vi "CheckWhetherSendMissions.vi"(10 "Mission Notifiers":T1, 11 "NotifierReff":T2) -> (2 "Send obstacles?":bool, 3 "Send missions?":bool)   [LabVIEW 2013]
doc: "This VI checks whether last the mission and obstacle ID held by the OCU matches that of the boat. If not, it signals that the missions need to be sent to the OCU to line the boat and OCU up again.\n\nEric Schneider, August 2014"
uses:
  Data/TypeDefs/Notifiers.ctl
  Data/TypeDefs/UTM Location.ctl
  Data/TypeDefs/Sail Set Suggestions.ctl
  Data/TypeDefs/Rudder Set Suggestions.ctl
  Data/TypeDefs/OverrideInformation.ctl
  Data/TypeDefs/OverrideMode.ctl
  Data/TypeDefs/MotorSetup.ctl
  Data/TypeDefs/DynamixelSetupInfo.ctl
  Data/TypeDefs/AirmarStatus.ctl
  Data/TypeDefs/HardwareOnline.ctl
  Data/TypeDefs/DynamixelCycleTracker.ctl
  Data/TypeDefs/RC Input Values.ctl
  Classes/Waypoint/Waypoint.lvclass
  Data/TypeDefs/MissionNotifiers.ctl
  Classes/Missions/GenericMission/GenericMission.lvclass
  Classes/Obstacle/Obstacle.lvclass
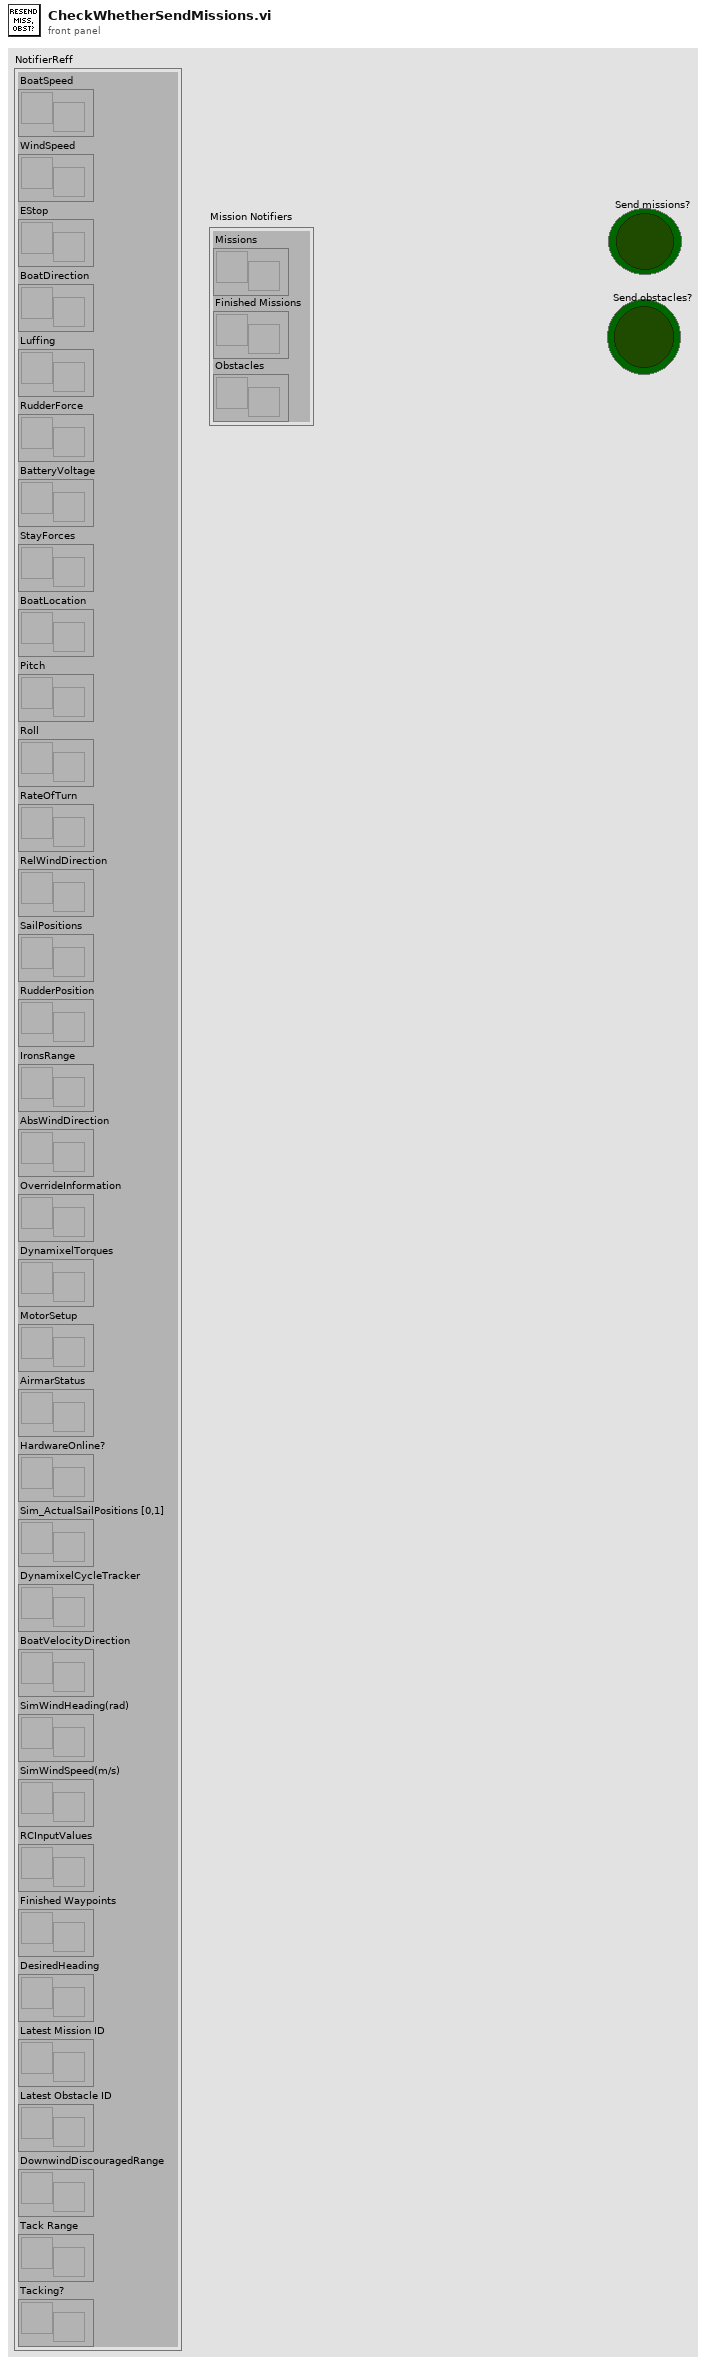
[diagram p1: front panel]
types:
  T1 = typedef "MissionNotifiers.ctl" = cluster{"Missions":refnum<notifier>, "Finished Missions":refnum<notifier>, "Obstacles":refnum<notifier>}
  T2 = typedef "Notifiers.ctl" = cluster{"BoatSpeed":refnum<notifier>, "WindSpeed":refnum<notifier>, "EStop":refnum<notifier>, "BoatDirection":refnum<notifier>, "Luffing":refnum<notifier>, "RudderForce":refnum<notifier>, "BatteryVoltage":refnum<notifier>, "StayForces":refnum<notifier>, "BoatLocation":refnum<notifier>, "Pitch":refnum<notifier>, "Roll":refnum<notifier>, "RateOfTurn":refnum<notifier>, "RelWindDirection":refnum<notifier>, "SailPositions":refnum<notifier>, "RudderPosition":refnum<notifier>, "IronsRange":refnum<notifier>, "AbsWindDirection":refnum<notifier>, "OverrideInformation":refnum<notifier>, "DynamixelTorques":refnum<notifier>, "MotorSetup":refnum<notifier>, "AirmarStatus":refnum<notifier>, "HardwareOnline?":refnum<notifier>, "Sim_ActualSailPositions [0,1]":refnum<notifier>, "DynamixelCycleTracker":refnum<notifier>, "BoatVelocityDirection":refnum<notifier>, "SimWindHeading(rad)":refnum<notifier>, "SimWindSpeed(m/s)":refnum<notifier>, "RCInputValues":refnum<notifier>, "Finished Waypoints":refnum<notifier>, "DesiredHeading":refnum<notifier>, "Latest Mission ID":refnum<notifier>, "Latest Obstacle ID":refnum<notifier>, "DownwindDiscouragedRange":refnum<notifier>, "Tack Range":refnum<notifier>, "Tacking?":refnum<notifier>}
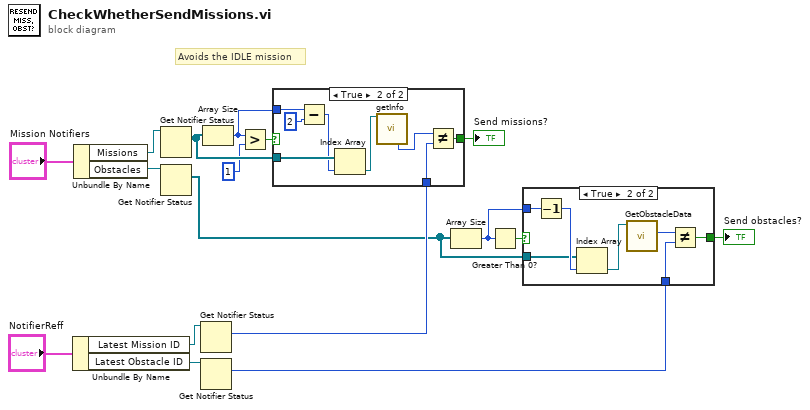
[diagram p0: block diagram]
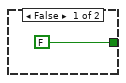
[diagram p2: hidden frame]
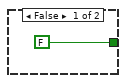
[diagram p3: hidden frame]
diagram:
  # "Avoids the IDLE mission"
  n1 = Unbundle By Name("NotifierReff") -> ("Latest Mission ID"=w11:refnum<notifier>, "Latest Obstacle ID"=w4:refnum<notifier>)
  n2 = Unbundle By Name("Mission Notifiers") -> ("Missions"=w16:refnum<notifier>, "Obstacles"=w15:refnum<notifier>)
  n3 = Get Notifier Status(notifier=w16) -> (current notification=w13:refnum<class "GenericMission.lvclass">[])  [unwired: 1 in, 4 out]
  n4 = Get Notifier Status(notifier=w15) -> (current notification=w5:refnum<class "Obstacle.lvclass">[])  [unwired: 1 in, 4 out]
  n5 = Get Notifier Status(notifier=w11) -> (current notification=w10:i32)  [unwired: 1 in, 4 out]
  n6 = Get Notifier Status(notifier=w4) -> (current notification=w9:i32)  [unwired: 1 in, 4 out]
  n7 = Array Size(array=w13) -> (size(s)=w3:i32)
  n8 = Greater?(x=w3, y=1) -> (0:w2:bool)
  n9 = case shown="True" w2 {
    tunnel: [FALSE w24] -> w14
    tunnel: w3 -> [_ w21]
    tunnel: w13 -> [_ w26]
    tunnel: w10 -> [_ w22]
    frame False {
    }
    frame True {
      n10 = Subtract(x=w21, y=2) -> (x-y=w20:i32)
      n11 = Index Array(array=w26, index=w20) -> (element=w25:refnum<class "GenericMission.lvclass">)
      n12 = call-dynamic "getInfo.vi"("GenericMission in"=w25) -> ("ID#"=w23:i16)  [unwired: 6 in, 8 out]
      n13 = Not Equal?(x=w23, y=w22) -> (x != y?=w24:bool)
    }
  }
  "Send missions?" <- w14
  n14 = Array Size(array=w5) -> (size(s)=w8:i32)
  n15 = Greater Than 0?(x=w8) -> (x > 0?=w6:bool)
  n16 = case shown="True" w6 {
    tunnel: [FALSE w32] -> w7
    tunnel: w8 -> [_ w34]
    tunnel: w9 -> [_ w31]
    tunnel: w5 -> [_ w30]
    frame False {
    }
    frame True {
      n17 = Decrement(x=w34) -> (x-1=w33:i32)
      n18 = Index Array(array=w30, index=w33) -> (element=w29:refnum<class "Obstacle.lvclass">)
      n19 = call "GetObstacleData.vi"("Obstacle.lvclass"=w29) -> ("ID#"=w28:i32)  [unwired: 7 in, 3 out]
      n20 = Not Equal?(x=w28, y=w31) -> (x != y?=w32:bool)
    }
  }
  "Send obstacles?" <- w7
